vi "TDT-Compute Skip Samples.vi"(0 "Device":T2, 5 "AO Fs (Hz)":dbl, 7 "Input":T1, 9 "AI Fs (Hz)":dbl) -> (8 "DO Samples":i32)   [LabVIEW 2020]
uses:
  Typedefs/TDT-Device ID.ctl
  Typedefs/TDT-Input source.ctl
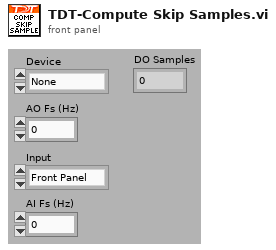
[diagram p1: front panel]
types:
  T1 = typedef "TDT-Input source.ctl" = enum16{"Front Panel", "RA4LI", "RA16LI"}
  T2 = typedef "TDT-Device ID.ctl" = enum16{"None", "PA5", "RP2", "RL2", "RA16", "RV8", "RX5", "RX6", "RX7", "RX8", "RZ2", "RZ5", "RZ6"}
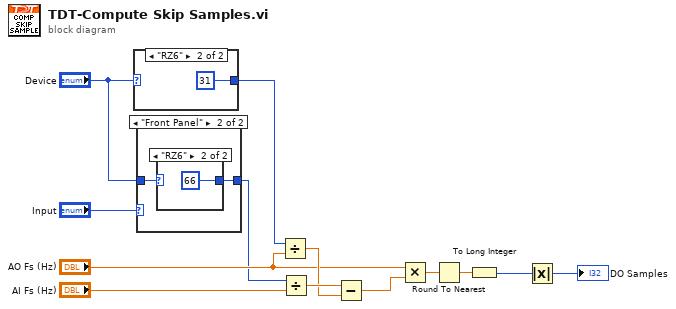
[diagram p0: block diagram]
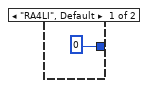
[diagram p2: hidden frame]
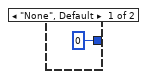
[diagram p3: hidden frame]
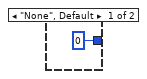
[diagram p4: hidden frame]
diagram:
  n1 = case shown="\"RZ6\"" "Device" {
    tunnel: [0 31] -> w13
    frame "None", Default {
    }
    frame "RZ6" {
    }
  }
  n2 = case shown="\"Front Panel\"" "Input" {
    tunnel: [0 w18] -> w3
    tunnel: "Device" -> [_ w17]
    frame "RA4LI", Default {
    }
    frame "Front Panel" {
      n3 = case shown="\"RZ6\"" w17 {
        tunnel: [0 66] -> w18
        frame "None", Default {
        }
        frame "RZ6" {
        }
      }
    }
  }
  n4 = Divide(x=w13, y="AO Fs (Hz)") -> (x/y=w10:dbl)
  n5 = Divide(x=w3, y="AI Fs (Hz)") -> (x/y=w11:dbl)
  n6 = Subtract(x=w11, y=w10) -> (x-y=w9:dbl)
  n7 = Multiply(x="AO Fs (Hz)", y=w9) -> (x*y=w7:dbl)
  n8 = Round To Nearest(number=w7) -> (nearest integer value=w6:dbl)
  n9 = To Long Integer(number=w6) -> (32bit integer=w5:i32)
  n10 = Absolute Value(x=w5) -> (abs(x)=→"DO Samples":i32)
